vi "APX VarianTMP GAS.vi"() -> ()   [LabVIEW 2015]
uses:
  <vilib>/Instr/_visa.llb/VISA Configure Serial Port (Instr).vi
  <userlib>/caLab/Private/Get_PV-1D.vi
  <userlib>/caLab/Private/Put_DBL-1D_PV-1D.vi
  <userlib>/caLab/Private/Put_DBL_PV.vi
panel:
  out "TMPC5STRSTP 2":string
  out "APX:GASTurboS":dbl
  out "element 2":dbl
  out "element":dbl
  out "SERIAL":string
  out "APX:GASTrubo_STOP":bool
  out "APX:GASTurbo_START":bool
  out "TMPC5STRSTP":string
  out "V-81":refnum<visa-resource-name>="COM4"
  out "APX:GASTurboF":dbl caption="F_20/Hz"
  out "APX:GASTurboP":dbl caption="P_20/W"
  out "APX:GASTurboS:STR":string
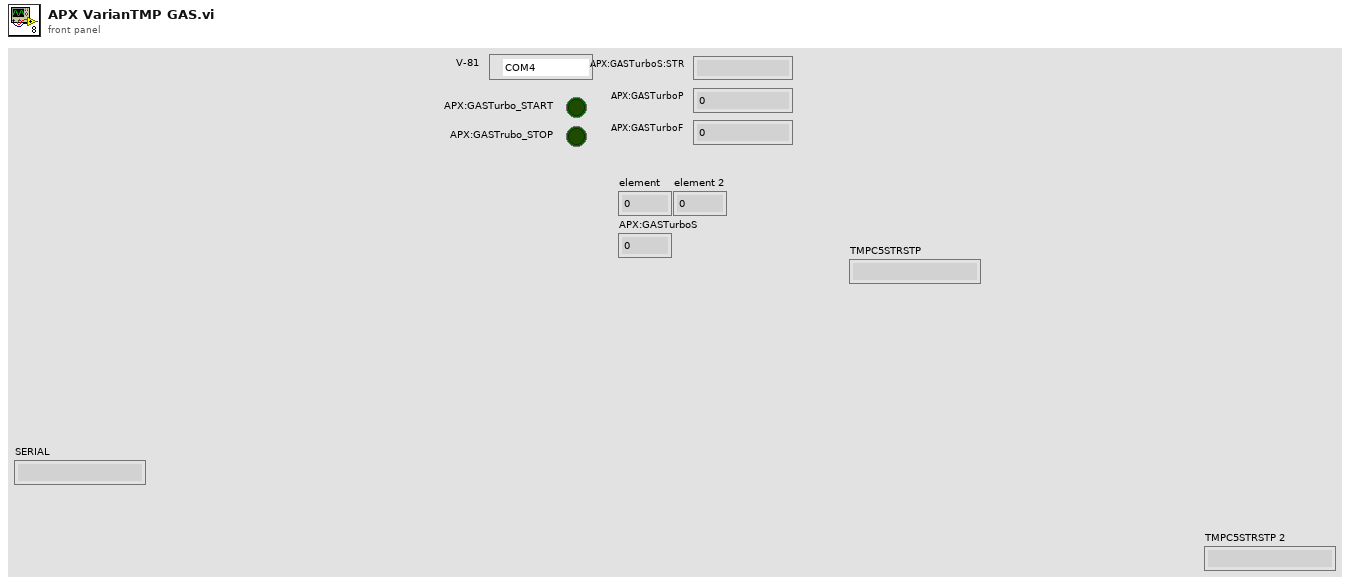
[diagram p1: front panel]
types:
  T1 = enum16{"START", "STOP", "REMOTE/SERIAL", "REMOTE", "SERIAL", "START/STOP", "PUMP STATUS", "Driving Frequency", "PUMP POWER", "PRESSURE"}
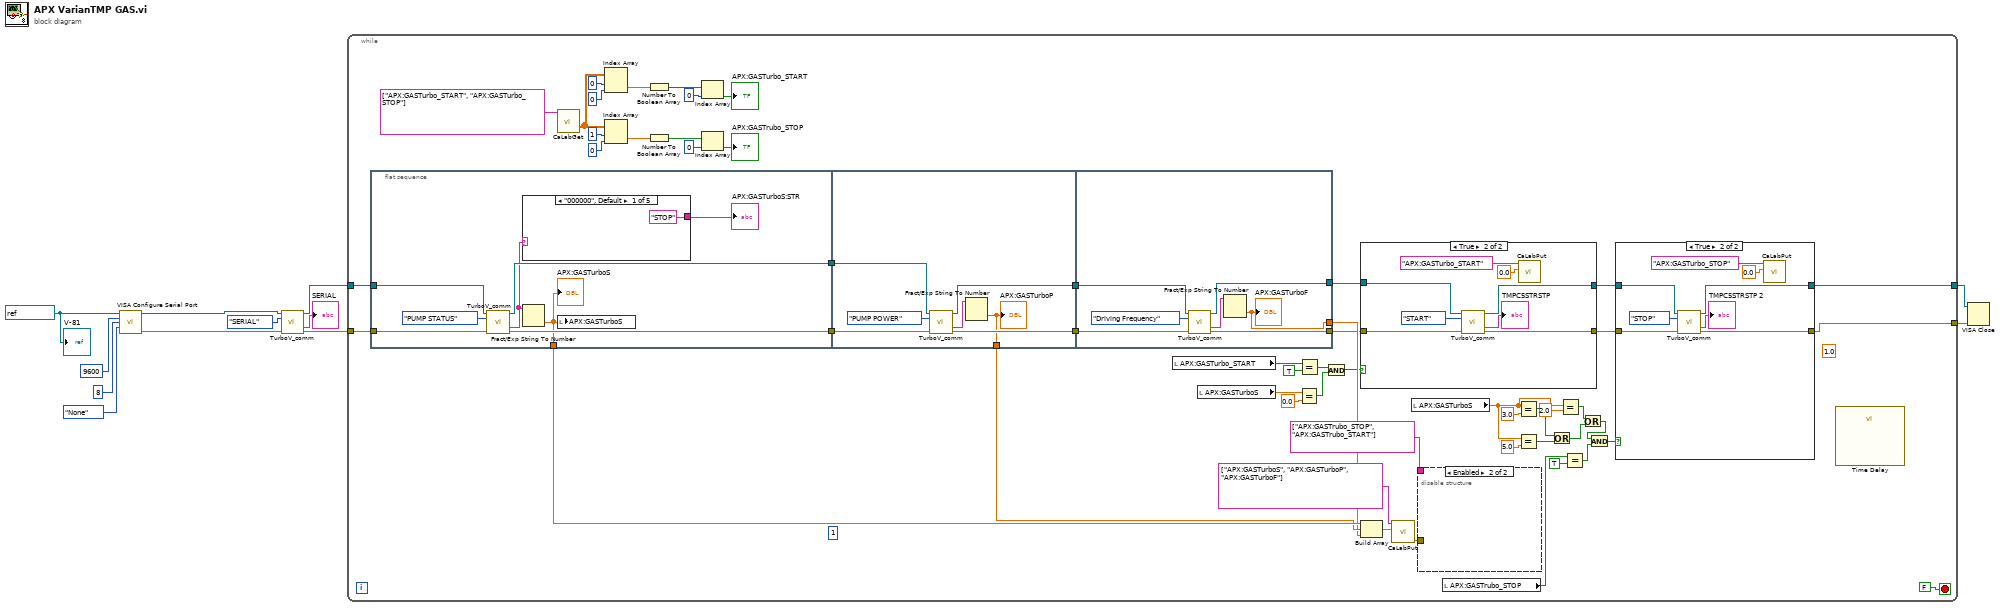
[diagram p0: block diagram]
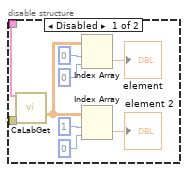
[diagram p2: hidden frame]
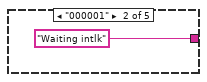
[diagram p3: hidden frame]
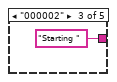
[diagram p4: hidden frame]
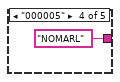
[diagram p5: hidden frame]
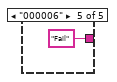
[diagram p6: hidden frame]
diagram:
  w12 = refnum<visa-resource-name> "COM26" ("VISA resource name")
  n1 = call-poly "VISA Configure Serial Port"("VISA resource name"=w12, "baud rate (9600)"=u32 9600, "data bits (8)"=u16 8, "parity (0:none)"=enum16{"None", "Odd", "Even", "Mark", "Space"}."None") -> ("VISA resource name out"=w4:refnum<visa-resource-name>, "error out"=w3:errorcluster)  [unwired: 10 in]
  n2 = call "TurboV_comm.vi"("VISA resource name"=w4, "Command"=T1."SERIAL", "error in (no error)"=w3) -> ("VISA resource name out"=w6:refnum<visa-resource-name>, "read buffer"=→"SERIAL":string, "error out"=w5:errorcluster)  [unwired: 10 in]
  n3 = while {
    tunnel: [w19] -> w8
    tunnel: w6 -> [w23]
    tunnel: w5 -> [w22]
    tunnel: [w18] -> w1
    stop <- FALSE stop-if-true
    (unwired) 1.0 ("Delay Time (s)")
    (unwired) 1
    n4 = flat-sequence {
      tunnel: [w83] -> w27
      tunnel: [w82] -> w26
      tunnel: [w78] -> w64
      tunnel: w23 -> [w77]
      tunnel: w22 -> [w76]
      tunnel: w27 -> [w94]
      tunnel: w26 -> [w91]
      tunnel: [w93] -> w25
      tunnel: [w92] -> w24
      tunnel: [w89] -> w63
      tunnel: w25 -> [w102]
      tunnel: w24 -> [w101]
      tunnel: [w98] -> w20
      tunnel: [w97] -> w21
      tunnel: [w96] -> w62
      frame #0 {
        n5 = call "TurboV_comm.vi"("VISA resource name"=w77, "Command"=T1."PUMP STATUS", "error in (no error)"=w76) -> ("VISA resource name out"=w83:refnum<visa-resource-name>, "read buffer"=w79:string, "error out"=w82:errorcluster)  [unwired: 10 in]
        n6 = case shown="\"000000\", Default" w79 {
          tunnel: ["STOP" "Waiting intlk" "Starting " "NOMARL" "Fail"] -> w80
          frame "000000", Default {
          }
          frame "000001" {
          }
          frame "000002" {
          }
          frame "000005" {
          }
          frame "000006" {
          }
        }
        "APX:GASTurboS:STR" <- w80
        n7 = Fract/Exp String To Number(string=w79) -> (number=w78:dbl)  [unwired: 3 in, 1 out]
        "APX:GASTurboS" <- w78
        n8 = local write "APX:GASTurboS"(w78) -> ()
      }
      frame #1 {
        n9 = call "TurboV_comm.vi"("VISA resource name"=w94, "Command"=T1."PUMP POWER", "error in (no error)"=w91) -> ("VISA resource name out"=w93:refnum<visa-resource-name>, "read buffer"=w90:string, "error out"=w92:errorcluster)  [unwired: 10 in]
        n10 = Fract/Exp String To Number(string=w90) -> (number=w89:dbl)  [unwired: 3 in, 1 out]
        "APX:GASTurboP" <- w89
      }
      frame #2 {
        n11 = call "TurboV_comm.vi"("VISA resource name"=w102, "Command"=T1."Driving Frequency", "error in (no error)"=w101) -> ("VISA resource name out"=w97:refnum<visa-resource-name>, "read buffer"=w99:string, "error out"=w98:errorcluster)  [unwired: 10 in]
        n12 = Fract/Exp String To Number(string=w99) -> (number=w96:dbl)  [unwired: 3 in, 1 out]
        "APX:GASTurboF" <- w96
      }
    }
    n13 = call-poly "CaLabGet.vi"("PV Names"=string[] ["APX:GASTurbo_START", "APX:GASTurbo_STOP"]) -> ("Value Array (number)"=w47:dbl[][])  [unwired: 8 in, 6 out]
    n14 = Index Array(array=w47, index (row)=0 ("disabled index (row)"), index (col)=0 ("index (row)")) -> (element=w53:dbl)
    n15 = Index Array(array=w47, index (row)=1 ("disabled index (row)"), index (col)=0 ("index (row)")) -> (element=w48:dbl)
    n16 = Number To Boolean Array(number=w53) -> (Boolean array=w55:bool[])
    n17 = Number To Boolean Array(number=w48) -> (Boolean array=w50:bool[])
    n18 = Index Array(array=w55, index=0) -> (element=→"APX:GASTurbo_START":bool)
    n19 = Index Array(array=w50, index=0) -> (element=→"APX:GASTrubo_STOP":bool)
    n20 = local read "APX:GASTurbo_START"() -> (w42:bool)
    n21 = local read "APX:GASTurboS"() -> (w43:dbl)
    n22 = Equal?(x=w43, y=0.0) -> (x = y?=w39:bool)
    n23 = Equal?(x=w42, y=TRUE) -> (x = y?=w40:bool)
    n24 = And(x=w40, y=w39) -> (x .and. y?=w38:bool)
    n25 = case shown="True" w38 {
      tunnel: [w114 w120] -> w33
      tunnel: [w113 w119] -> w32
      tunnel: w21 -> [w114 w118]
      tunnel: w20 -> [w113 w117]
      frame False {
      }
      frame True {
        n26 = call "TurboV_comm.vi"("VISA resource name"=w118, "Command"=T1."START", "error in (no error)"=w117) -> ("VISA resource name out"=w120:refnum<visa-resource-name>, "read buffer"=→"TMPC5STRSTP":string, "error out"=w119:errorcluster)  [unwired: 10 in]
        n27 = call-poly <userlib>:"CaLabPut.vi"("Value"=0.0, "PV Name"="APX:GASTurbo_START") -> ()  [unwired: 6 in, 4 out]
      }
    }
    n28 = Build Array(w64, w63, w62) -> (w61:dbl[])
    n29 = call-poly <userlib>:"CaLabPut.vi"("Values"=w61, "PV Names"=string[] ["APX:GASTurboS", "APX:GASTurboP", "APX:GASTurboF"]) -> ("Error out"=w59:errorcluster)  [unwired: 6 in, 3 out]
    n30 = local read "APX:GASTurboS"() -> (w17:dbl)
    n31 = disable-structure shown="Enabled" {
      disable-tunnel: string[] ["APX:GASTrubo_STOP", "APX:GASTrubo_START"] -> [w75 _]
      disable-tunnel: w59 -> [w74 _]
      frame Disabled {
        n32 = call-poly "CaLabGet.vi"("PV Names"=w75, "Error in (no error)"=w74) -> ("Value Array (number)"=w72:dbl[][])  [unwired: 7 in, 6 out]
        n33 = Index Array(array=w72, index (row)=0 ("disabled index (col)"), index (col)=0) -> (element=→"element":dbl)
        n34 = Index Array(array=w72, index (row)=1, index (col)=0) -> (element=→"element 2":dbl)
      }
      frame Enabled {
      }
    }
    n35 = local read "APX:GASTrubo_STOP"() -> (w29:bool)
    n36 = Equal?(x=w17, y=3.0) -> (x = y?=w35:bool)
    n37 = Equal?(x=w17, y=5.0) -> (x = y?=w34:bool)
    n38 = Or(x=w35, y=w34) -> (x .or. y?=w14:bool)
    n39 = Equal?(x=w17, y=2.0) -> (x = y?=w15:bool)
    n40 = Equal?(x=w29, y=TRUE) -> (x = y?=w30:bool)
    n41 = Or(x=w15, y=w14) -> (x .or. y?=w13:bool)
    n42 = And(x=w13, y=w30) -> (x .and. y?=w31:bool)
    n43 = case shown="True" w31 {
      tunnel: [w104 w111] -> w19
      tunnel: [w103 w110] -> w18
      tunnel: w33 -> [w104 w108]
      tunnel: w32 -> [w103 w107]
      frame False {
      }
      frame True {
        n44 = call "TurboV_comm.vi"("VISA resource name"=w108, "Command"=T1."STOP", "error in (no error)"=w107) -> ("VISA resource name out"=w111:refnum<visa-resource-name>, "read buffer"=→"TMPC5STRSTP 2":string, "error out"=w110:errorcluster)  [unwired: 10 in]
        n45 = call-poly <userlib>:"CaLabPut.vi"("Value"=0.0, "PV Name"="APX:GASTurbo_STOP") -> ()  [unwired: 6 in, 4 out]
      }
    }
    n46 = call "Time Delay"() -> ()  [unwired: 11 in, 1 out]
  }
  n47 = VISA Close(VISA resource name=w8, error in (no error)=w1) -> ()  [unwired: 1 out]
  "V-81" <- w12
